vi "BDSCTRL_Main.vi"() -> ()   [LabVIEW 2016]
uses:
  BDSCTRL_Controls/BDSCTRL_Panel_Action_List.ctl
  BDSCTRL_Controls/BDSCTRL_Panel_Poll_Function_List.ctl
  BDSCTRL_Globals/BDSCTRL_Global_Working_Directory.vi
panel:
  in  "error in \n(no error)":errorcluster
  out "Working Directory":path
  in  "stop":bool
  in  "Digital Gain":dbl
  in  "Test Status":string="Awaiting User Selection..."
  in  "Tab Control":T1(tab)
  in  "DMA Settings Cluster":T2
  in  "MB-CFR Settings Cluster":T3
  in  "Set Beam Settings Cluster":T4
  in  "RF Parameters Settings Cluster":T5={"RF Bandwidth \n(MHz)"=0, "Tx RF \nFrequency"=2132.5, "Tx VGA"=[], "Rx VGA"=[]}
  in  "Target Devices":T6={"P1 Cluster"={"P1_D1"=TRUE, "P1_D2"=TRUE, "P1_D3"=TRUE, "P1_D4"=TRUE, "P1_D5"=TRUE, "P1_D6"=TRUE, "P1_D7"=TRUE, "P1_D8"=TRUE, "P1_D9"=TRUE, "P1_D10"=TRUE, "P1_D11"=TRUE, "P1_D12"=TRUE, "P1_D13"=TRUE, "P1_D14"=TRUE, "P1_D15"=TRUE, "P1_D16"=TRUE, "P1_D17"=TRUE, "P1_D18"=TRUE, "P1_D19"=TRUE, "P1_D20"=TRUE, "P1_D21"=TRUE, "P1_D22"=TRUE, "P1_D23"=TRUE, "P1_D24"=TRUE}, "P2 Cluster"={"P2_D1"=TRUE, "P2_D2"=TRUE, "P2_D3"=TRUE, "P2_D4"=TRUE, "P2_D5"=TRUE, "P2_D6"=TRUE, "P2_D7"=TRUE, "P2_D8"=TRUE, "P2_D9"=TRUE, "P2_D10"=TRUE, "P2_D11"=TRUE, "P2_D12"=TRUE, "P2_D13"=TRUE, "P2_D14"=TRUE, "P2_D15"=TRUE, "P2_D16"=TRUE, "P2_D17"=TRUE, "P2_D18"=TRUE, "P2_D19"=TRUE, "P2_D20"=TRUE, "P2_D21"=TRUE, "P2_D22"=TRUE, "P2_D23"=TRUE, "P2_D24"=TRUE}}
  in  "Polling Enable":bool
  in  "Polling Functions":T7
  in  "Read Polling Function":bool
  in  "Query Poll Function":T8
  in  "Exe Panel Action":bool
  in  "Panel Action":T9 items=["Panel Init", "RF Calibration", "Rotate Beam", "Set RF Frequency", "Initial Calibrations", "Channel Enable", "IF Calibration", "Sense Power", "Measure Temperature", "Set RF Power Level", "Run DMA", "Set RF Bandwidth", "Set CFR", "Set Beam"]
  in  "Exe Panel Action Sequence":bool
  in  "Panel Action Sequence":T9[](array[typedef]) items=["Panel Init", "RF Calibration", "Rotate Beam", "Set RF Frequency", "Initial Calibrations", "Channel Enable", "IF Calibration", "Sense Power", "Measure Temperature", "Set RF Power Level", "Run DMA", "Set RF Bandwidth", "Set CFR", "Set Beam"]
  in  "Beam Rotation":string[][](table)=[["1"], ["1"], ["1"], ["1"], ["1"], ["1"], ["2"], ["2"], ["2"], ["2"], ["2"], ["2"]]
  in  "Target String":string="{1:24,1:24,[],[]}"
  in  "Update Targets":bool
  in  "Channels Cluster":T10={"TX1"=TRUE, "TX2"=TRUE, "TX3"=FALSE, "TX4"=FALSE, "TXx3"=TRUE, "TXx4"=TRUE, "RX1"=FALSE, "RX2"=FALSE, "RX3"=FALSE, "RX4"=FALSE, "RXx3"=FALSE, "RXx4"=FALSE, "Tx"=TRUE, "Rx"=FALSE}
  in  "Test List Cluster":T11={"Test List"=[{"Test Process"=enum."Sanity Check", "Update Targets 3"=FALSE, "Enable"=TRUE}, {"Test Process"=enum."Power Accuracy", "Update Targets 3"=FALSE, "Enable"=TRUE}, {"Test Process"=enum."ACLR", "Update Targets 3"=FALSE, "Enable"=TRUE}, {"Test Process"=enum."EVM", "Update Targets 3"=FALSE, "Enable"=TRUE}, {"Test Process"=enum."Rx Sensitivity", "Update Targets 3"=FALSE, "Enable"=TRUE}, {"Test Process"=enum."Scan Beam", "Update Targets 3"=FALSE, "Enable"=TRUE}], "Execute List"=FALSE, "RF Settings List"=[{"RF Bandwidth \n(MHz)"=10, "Tx Frequency \n(MHz)"=2115.0, "TX Attenuation"=[51, 51, 51, 51], "RX Attenuation"=[20, 20, 20, 20], "RF Settings List: Channel Cluster"={"TX1 2"=TRUE, "TX1 3"=TRUE, "TX1 4"=FALSE, "TX1 5"=FALSE, "TX1 6"=TRUE, "TX1 7"=TRUE, "TX1"=FALSE, "TX1 8"=FALSE, "TX1 9"=FALSE, "TX1 10"=FALSE, "TX1 11"=FALSE, "TX1 12"=FALSE, "Tx"=TRUE, "Rx"=FALSE}}, {"RF Bandwidth \n(MHz)"=10, "Tx Frequency \n(MHz)"=2132.5, "TX Attenuation"=[63, 63, 63, 63], "RX Attenuation"=[63, 63, 63, 63], "RF Settings List: Channel Cluster"={"TX1 2"=TRUE, "TX1 3"=TRUE, "TX1 4"=FALSE, "TX1 5"=FALSE, "TX1 6"=TRUE, "TX1 7"=TRUE, "TX1"=FALSE, "TX1 8"=FALSE, "TX1 9"=FALSE, "TX1 10"=FALSE, "TX1 11"=FALSE, "TX1 12"=FALSE, "Tx"=TRUE, "Rx"=FALSE}}]}
  in  "Configure Manual Test":bool
  in  "Test Process":T12(ring)=enum."Scan Beam"
  in  "Execute Test":bool
  in  "Save Settings":bool
  in  "Load Settings":bool
  in  "MXG Test Connection":bool
  in  "EXA Test Connection":bool
  in  "Melvitron Test Connection":bool
  in  "Panel IP Address":string="10.1.11.247"
  in  "EXA IP Address":string="10.1.11.123"
  in  "MXG IP Address":string="10.1.11.122"
  in  "Melvitron IP Address":string="COM12"
  in  "Panel Test Connection":bool
  in  "Test Setup Settings Cluster":T13={"IF Calibration File"=path "IFCalExample.csv", "Beam Lookup Table"=path "BeamLookupTableExample.csv", "Test Environment"=enum."Melvitron", "Panel Mode"=enum."CPRI", "Calibration Mode"=0, "Panel Type"=0, "Band"=0, "Tile"=0, " API Drop"=0} {"API Drop" items=["MAY", "JUNE"]; "Tile" items=["HP-C", "HP-B3"]; "Band" items=["AWS", "PCS-A", "PCS-G"]; "Panel Type" items=["Half", "Full", "Quarter"]; "Calibration Mode" items=["Manual", "SemiAuto", "Auto"]}
  out "SW Version":string
  # "Most useful Panel Status info in common region"
  # "Panel Selections"
  # "Panel Action Settings"
  # "Polling Functions"
  # "Panel Action Execution"
  # "DMA"
  # "MB-CFR"
  # "Set Beam"
  # "RF Parameters"
  # "P2"
  # "P1"
  # "Auto Polling"
  # "Period (s)"
  # "Manual Polling"
  # "Manual Test Process"
  # "Test Connection"
  # "Similar to Panel Status GUI/Window"
  # "Show Results summary from each completed test"
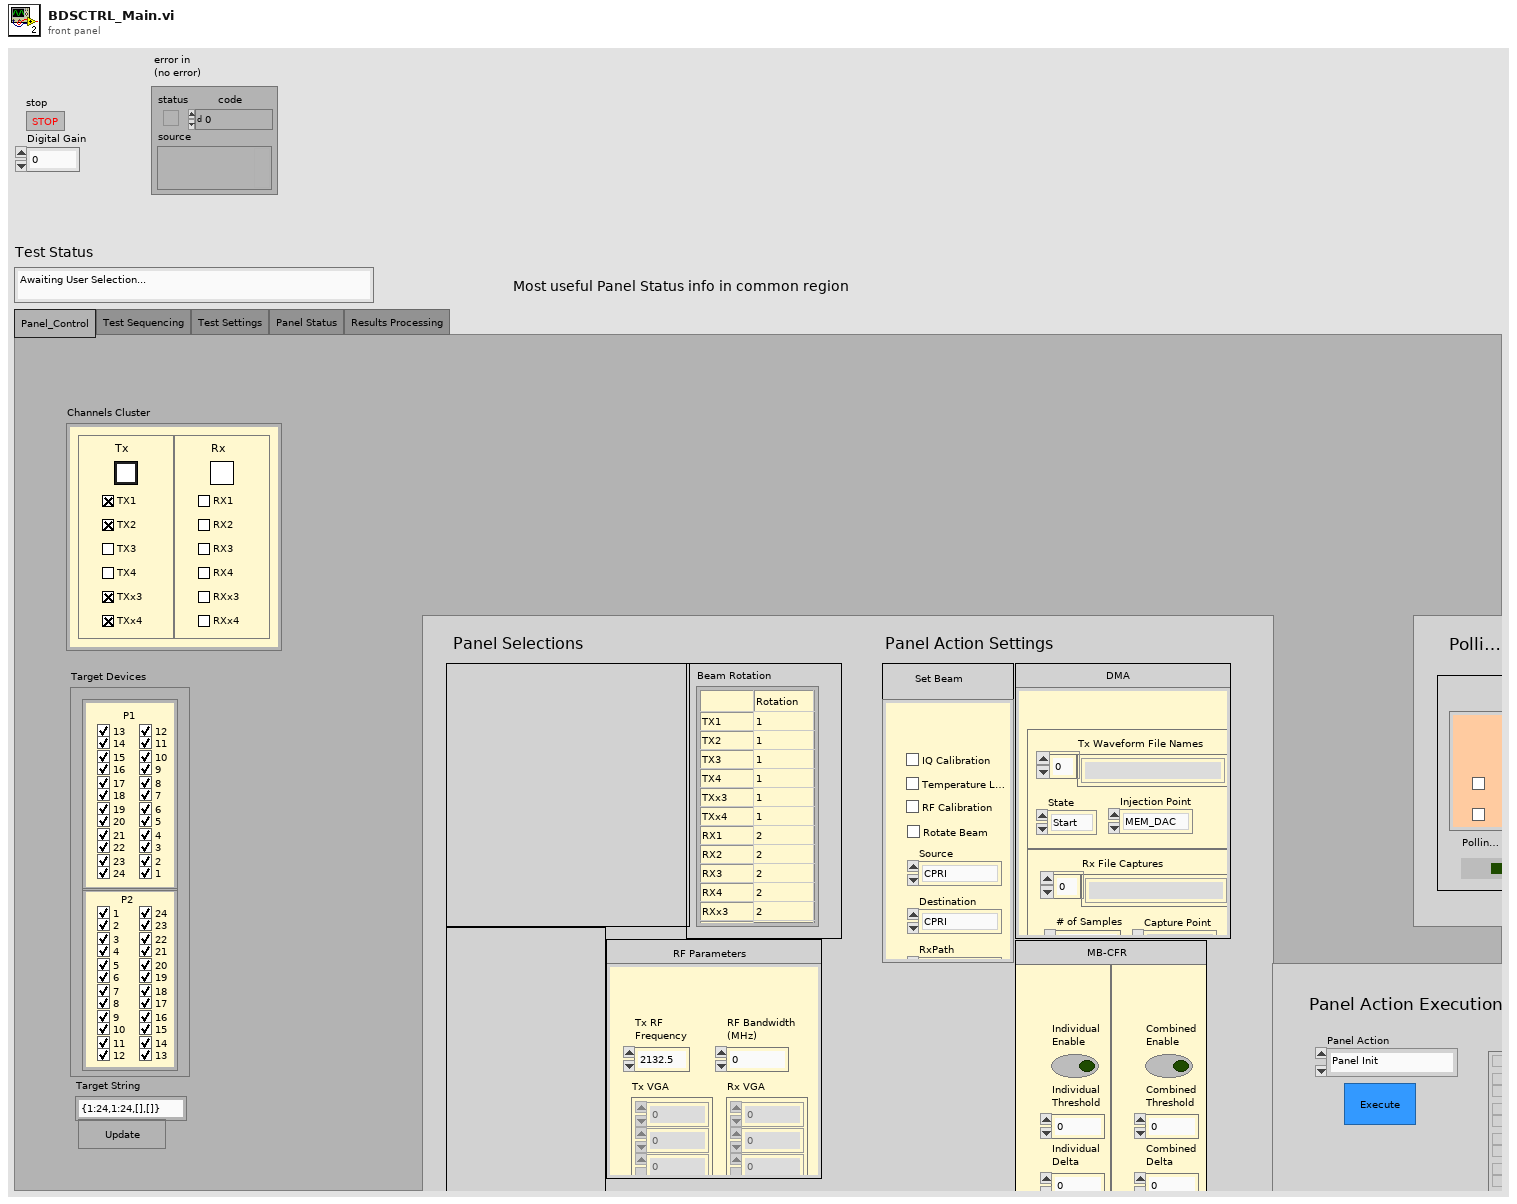
[diagram p1: front panel]
types:
  T1 = enum32{"Panel_Control", "Test Sequencing", "Test Settings", "Panel Status", "Results Processing"}
  T2 = cluster{"Tx Waveform File Names":string[], "State":enum16{"Start", "Stop"}, "Injection Point":enum16{"MEM_DAC", "MEM_DUC"}, "Rx File Captures":string[], "# of Samples":i32, "Capture Point":enum16{"MEM_ADC", "MEM_DDC"}}
  T3 = cluster{"Individual\nEnable":bool, "Individual\nThreshold":dbl, "Individual\nDelta":dbl, "Individual\nWeight":dbl, "Combined\nEnable":bool, "Combined\nThreshold":dbl, "Combined\nDelta":dbl}
  T4 = cluster{"IQ Calibration":bool, "Temperature Loop":bool, "RF Calibration":bool, "Rotate Beam":bool, "Source":enum16{"CPRI", "CAL", "MEM_DAC", "MEM_DUC", "EXT"}, "Destination":enum16{"CPRI", "EXT", "MEM_ADC", "MEM_DDC"}, "RxPath":enum16{"DIRECT", "MIXER"}}
  T5 = cluster{"RF Bandwidth \n(MHz)":i32, "Tx RF \nFrequency":dbl, "Tx VGA":i32[], "Rx VGA":i32[]}
  T6 = cluster{"P1 Cluster":cluster{"P1_D1":bool, "P1_D2":bool, "P1_D3":bool, "P1_D4":bool, "P1_D5":bool, "P1_D6":bool, "P1_D7":bool, "P1_D8":bool, "P1_D9":bool, "P1_D10":bool, "P1_D11":bool, "P1_D12":bool, "P1_D13":bool, "P1_D14":bool, "P1_D15":bool, "P1_D16":bool, "P1_D17":bool, "P1_D18":bool, "P1_D19":bool, "P1_D20":bool, "P1_D21":bool, "P1_D22":bool, "P1_D23":bool, "P1_D24":bool}, "P2 Cluster":cluster{"P2_D1":bool, "P2_D2":bool, "P2_D3":bool, "P2_D4":bool, "P2_D5":bool, "P2_D6":bool, "P2_D7":bool, "P2_D8":bool, "P2_D9":bool, "P2_D10":bool, "P2_D11":bool, "P2_D12":bool, "P2_D13":bool, "P2_D14":bool, "P2_D15":bool, "P2_D16":bool, "P2_D17":bool, "P2_D18":bool, "P2_D19":bool, "P2_D20":bool, "P2_D21":bool, "P2_D22":bool, "P2_D23":bool, "P2_D24":bool}}
  T7 = cluster{"Boolean 6":bool, "Boolean 7":bool, "Boolean 9":bool, dbl, dbl, dbl}
  T8 = typedef "BDSCTRL_Panel_Poll_Function_List.ctl" = enum16{"DFE Info", "DFE Electrical", "DFE Clock", "DFE CPRI", "DFE Temp", "DFE RF Power", "Tile Temperature", "Tile SPI", "Tile Info", "Tile RF Power", "Tile PLL Lock", "Tile PA Linearization", "Tile PA Bias"}
  T9 = typedef "BDSCTRL_Panel_Action_List.ctl" = u16
  T10 = cluster{"TX1":bool, "TX2":bool, "TX3":bool, "TX4":bool, "TXx3":bool, "TXx4":bool, "RX1":bool, "RX2":bool, "RX3":bool, "RX4":bool, "RXx3":bool, "RXx4":bool, "Tx":bool, "Rx":bool}
  T11 = cluster{"Test List":cluster{"Test Process":enum16{"Set Beam", "Scan Beam", "Sanity Check", "Power Accuracy", "ACLR", "EVM", "Rx Sensitivity"}, "Update Targets 3":bool, "Enable":bool}[], "Execute List":bool, "RF Settings List":cluster{"RF Bandwidth \n(MHz)":i32, "Tx Frequency \n(MHz)":dbl, "TX Attenuation":i32[], "RX Attenuation":i32[], "RF Settings List: Channel Cluster":cluster{"TX1 2":bool, "TX1 3":bool, "TX1 4":bool, "TX1 5":bool, "TX1 6":bool, "TX1 7":bool, "TX1":bool, "TX1 8":bool, "TX1 9":bool, "TX1 10":bool, "TX1 11":bool, "TX1 12":bool, "Tx":bool, "Rx":bool}}[]}
  T12 = enum16{"Set Beam", "Scan Beam", "Sanity Check", "Power Accuracy", "ACLR", "EVM", "Rx Sensitivity"}
  T13 = cluster{"IF Calibration File":path, "Beam Lookup Table":path, "Test Environment":enum16{"Melvitron", "Spider", "Marinotron"}, "Panel Mode":enum16{"CPRI", "UpDnCnv"}, "Calibration Mode":u16, "Panel Type":u16, "Band":u16, "Tile":u16, " API Drop":u16}
  T14 = cluster{"Target Devices":cluster{"P1 Cluster":cluster{"P1_D1":bool, "P1_D2":bool, "P1_D3":bool, "P1_D4":bool, "P1_D5":bool, "P1_D6":bool, "P1_D7":bool, "P1_D8":bool, "P1_D9":bool, "P1_D10":bool, "P1_D11":bool, "P1_D12":bool, "P1_D13":bool, "P1_D14":bool, "P1_D15":bool, "P1_D16":bool, "P1_D17":bool, "P1_D18":bool, "P1_D19":bool, "P1_D20":bool, "P1_D21":bool, "P1_D22":bool, "P1_D23":bool, "P1_D24":bool}, "P2 Cluster":cluster{"P2_D1":bool, "P2_D2":bool, "P2_D3":bool, "P2_D4":bool, "P2_D5":bool, "P2_D6":bool, "P2_D7":bool, "P2_D8":bool, "P2_D9":bool, "P2_D10":bool, "P2_D11":bool, "P2_D12":bool, "P2_D13":bool, "P2_D14":bool, "P2_D15":bool, "P2_D16":bool, "P2_D17":bool, "P2_D18":bool, "P2_D19":bool, "P2_D20":bool, "P2_D21":bool, "P2_D22":bool, "P2_D23":bool, "P2_D24":bool}}, "Target String":string}
  T15 = cluster{"Tx RF \nFrequency":dbl, "RF Bandwidth \n(MHz)":i32, "Tx VGA":i32[], "Rx VGA":i32[]}
  T16 = cluster{"Panel IP Address":string, "Melvitron IP Address":string, "EXA IP Address":string, "MXG IP Address":string}
  T17 = cluster{"IF Calibration File":path, "Beam Lookup Table":path, "Test Environment":enum16{"Melvitron", "Spider", "Marinotron"}, "Panel Mode":enum16{"CPRI", "UpDnCnv"}, "Calibration Mode":u16, "Panel Type":u16, "Band":u16, "Tile":u16, "API Drop":u16}
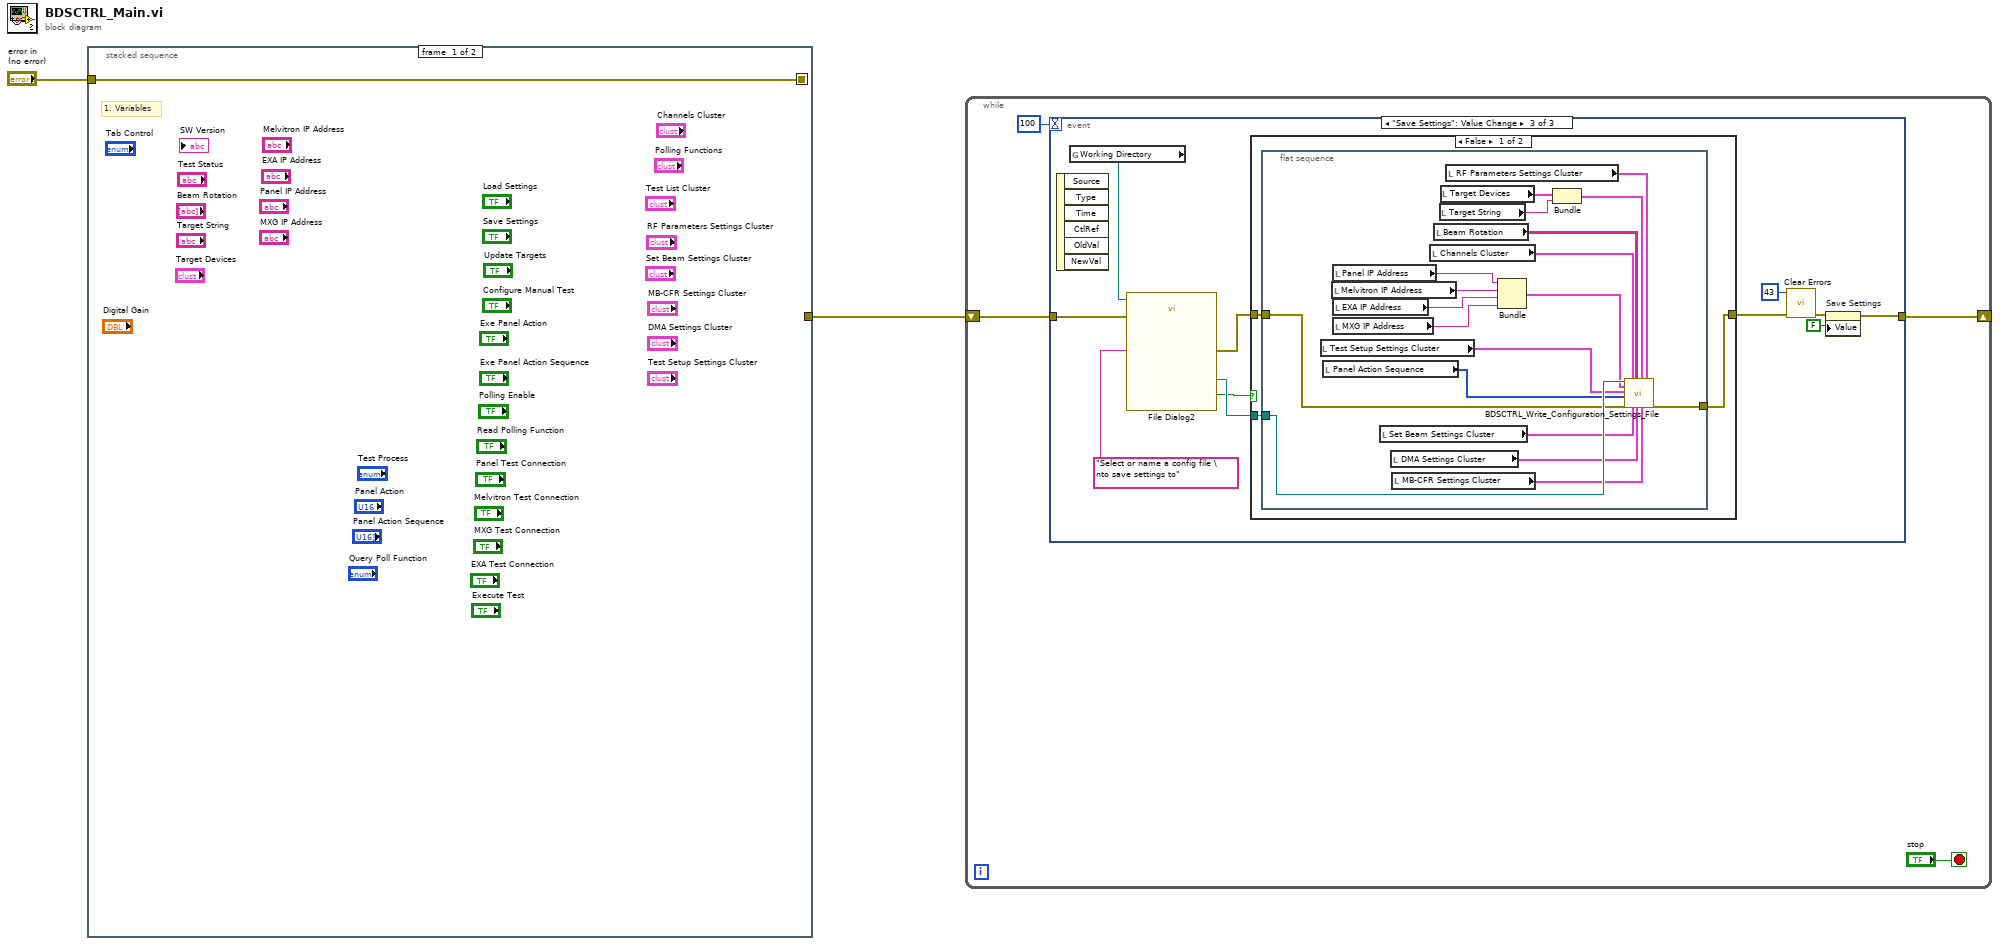
[diagram p0: block diagram]
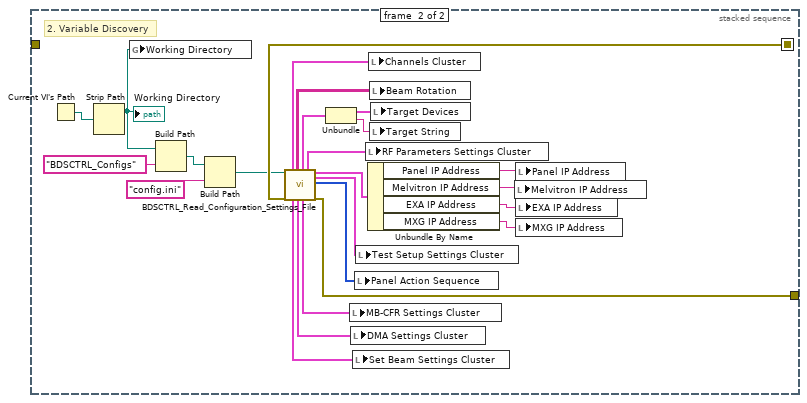
[diagram p2: hidden frame]
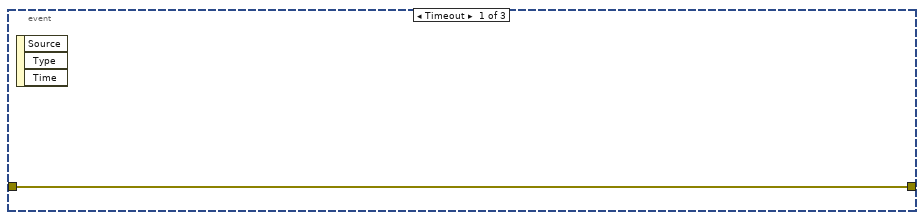
[diagram p3: hidden frame]
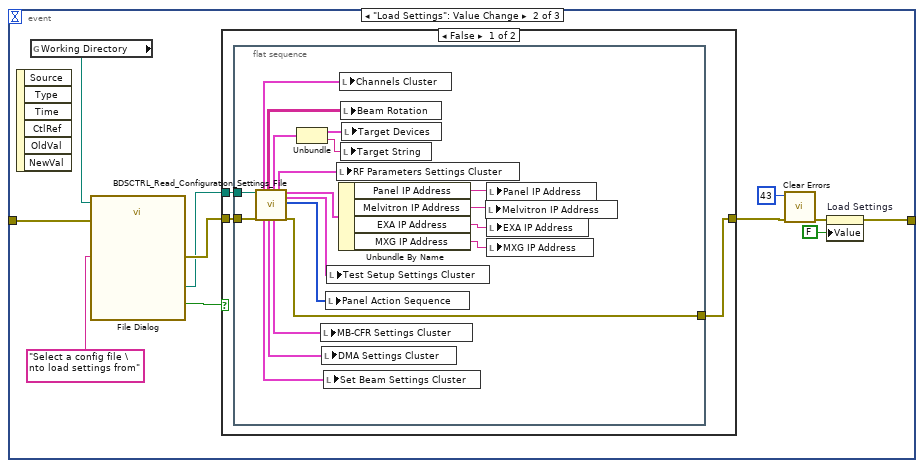
[diagram p4: hidden frame]
diagram:
  n1 = stacked-sequence {
    seq-local: [w3 _] -> [_ w26]
    tunnel: "error in \n(no error)" -> [w3 _]
    tunnel: [_ w6] -> w1
    frame #0 {
      # "1. Variables"
    }
    frame #1 {
      # "2. Variable Discovery"
      n2 = Current VI's Path() -> (path=w27:path)
      n3 = Strip Path(path=w27) -> (stripped path=w25:path)  [unwired: 1 out]
      "Working Directory" <- w25
      n4 = global write "BDSCTRL_Global_Working_Directory.vi" "Working Directory"(w25) -> ()
      n5 = Build Path(base path=w25, name or relative path="BDSCTRL_Configs") -> (appended path=w23:path)
      n6 = Build Path(base path=w23, name or relative path="config.ini") -> (appended path=w21:path)
      n7 = call "BDSCTRL_Read_Configuration_Settings_File.vi"("configuration file path"=w21, "error in \n(no error)"=w26) -> ("Channels Cluster"=w15:T10, "Set Beam Settings Cluster"=w4:T4, "Beam Rotation"=w19:string[][], "DMA Settings Cluster"=w5:T2, "Target Devices Settings Cluster"=w18:T14, "MB-CFR Settings Cluster"=w7:T3, "RF Parameters Settings Cluster"=w20:T15, "BDSCTRL Connection Settings"=w14:T16, "Test Setup Settings"=w9:T17, "Panel Action Sequence"=w8:T9[], "error out"=w6:errorcluster)  [unwired: 7 in]
      n8 = Unbundle(w18) -> ("Target Devices"=w17:T6, "Target String"=w16:string)
      n9 = local write "MB-CFR Settings Cluster"(w7) -> ()
      n10 = local write "DMA Settings Cluster"(w5) -> ()
      n11 = local write "Set Beam Settings Cluster"(w4) -> ()
      n12 = local write "Panel Action Sequence"(w8) -> ()
      n13 = local write "Test Setup Settings Cluster"(w9) -> ()
      n14 = local write "RF Parameters Settings Cluster"(w20) -> ()
      n15 = Unbundle By Name(w14) -> ("Panel IP Address"=w13:string, "Melvitron IP Address"=w12:string, "EXA IP Address"=w11:string, "MXG IP Address"=w10:string)
      n16 = local write "Channels Cluster"(w15) -> ()
      n17 = local write "Beam Rotation"(w19) -> ()
      n18 = local write "Target String"(w16) -> ()
      n19 = local write "Target Devices"(w17) -> ()
      n20 = local write "Melvitron IP Address"(w12) -> ()
      n21 = local write "Panel IP Address"(w13) -> ()
      n22 = local write "EXA IP Address"(w11) -> ()
      n23 = local write "MXG IP Address"(w10) -> ()
    }
  }
  n24 = while {
    shift-right: [w28] -> _
    shift-left: w1 -> [w29]
    stop <- "stop" stop-if-true
    n25 = event shown="[2] \"Save Settings\": Value Change" {
      selector: _ -> [_ _ _]
      dyn-events: _ -> [_ _ _]
      timeout: 100 -> [_ _ _]
      tunnel: w29 -> [w32 w39 w73]
      tunnel: [w32 w38 w71] -> w28
      event Timeout {
        n26 = event-data() -> ()  [unwired: 1 in, 3 out]
      }
      event "Load Settings": Value Change {
        n27 = event-data() -> ()  [unwired: 1 in, 6 out]
        n28 = global read "BDSCTRL_Global_Working_Directory.vi" "Working Directory"() -> (w43:path)
        n29 = call "File Dialog"("start path"=w43, "prompt"="Select a config file \nto load settings from", "error in"=w39) -> ("selected path"=w41:path, "cancelled"=w40:bool, "error out"=w42:errorcluster)  [unwired: 9 in, 1 out]
        n30 = case shown="False" w40 {
          tunnel: w42 -> [w46 w66]
          tunnel: w41 -> [w45 _]
          tunnel: [w44 w66] -> w34
          frame False {
            n31 = flat-sequence {
              tunnel: w46 -> [w49]
              tunnel: w45 -> [w48]
              tunnel: [w47] -> w44
              frame #0 {
                n32 = call "BDSCTRL_Read_Configuration_Settings_File.vi"("configuration file path"=w48, "error in \n(no error)"=w49) -> ("Channels Cluster"=w55:T10, "Set Beam Settings Cluster"=w65:T4, "Beam Rotation"=w51:string[][], "DMA Settings Cluster"=w64:T2, "Target Devices Settings Cluster"=w52:T14, "MB-CFR Settings Cluster"=w63:T3, "RF Parameters Settings Cluster"=w50:T15, "BDSCTRL Connection Settings"=w56:T16, "Test Setup Settings"=w61:T17, "Panel Action Sequence"=w62:T9[], "error out"=w47:errorcluster)  [unwired: 7 in]
                n33 = Unbundle(w52) -> ("Target Devices"=w53:T6, "Target String"=w54:string)
                n34 = local write "MB-CFR Settings Cluster"(w63) -> ()
                n35 = local write "DMA Settings Cluster"(w64) -> ()
                n36 = local write "Set Beam Settings Cluster"(w65) -> ()
                n37 = local write "Panel Action Sequence"(w62) -> ()
                n38 = local write "Test Setup Settings Cluster"(w61) -> ()
                n39 = local write "RF Parameters Settings Cluster"(w50) -> ()
                n40 = Unbundle By Name(w56) -> ("Panel IP Address"=w57:string, "Melvitron IP Address"=w58:string, "EXA IP Address"=w59:string, "MXG IP Address"=w60:string)
                n41 = local write "Channels Cluster"(w55) -> ()
                n42 = local write "Beam Rotation"(w51) -> ()
                n43 = local write "Target String"(w54) -> ()
                n44 = local write "Target Devices"(w53) -> ()
                n45 = local write "Melvitron IP Address"(w58) -> ()
                n46 = local write "Panel IP Address"(w57) -> ()
                n47 = local write "EXA IP Address"(w59) -> ()
                n48 = local write "MXG IP Address"(w60) -> ()
              }
            }
          }
          frame True {
          }
        }
        n49 = call <vilib>:"Clear Errors.vi"("error in (no error)"=w34, "specific error code to clear (0: all)"=43) -> ("error out"=w33:errorcluster)  [unwired: 4 in, 1 out]
        n50 = property on="Load Settings" class="Bool (strict)"(error in=w33, "Value"=FALSE ("Load Settings")) -> (error out=w38:errorcluster)  [unwired: 1 in, 1 out]
      }
      event "Save Settings": Value Change {
        n51 = event-data() -> ()  [unwired: 1 in, 6 out]
        n52 = global read "BDSCTRL_Global_Working_Directory.vi" "Working Directory"() -> (w77:path)
        n53 = call "File Dialog2"("start path"=w77, "prompt"="Select or name a config file \nto save settings to", "error in"=w73) -> ("selected path"=w75:path, "cancelled"=w74:bool, "error out"=w76:errorcluster)  [unwired: 9 in, 1 out]
        n54 = case shown="False" w74 {
          tunnel: w76 -> [w80 w100]
          tunnel: w75 -> [w79 _]
          tunnel: [w78 w100] -> w69
          frame False {
            n55 = flat-sequence {
              tunnel: w80 -> [w81]
              tunnel: w79 -> [w88]
              tunnel: [w99] -> w78
              frame #0 {
                n56 = local read "Test Setup Settings Cluster"() -> (w86:T13)
                n57 = local read "Panel Action Sequence"() -> (w85:T9[])
                n58 = local read "Melvitron IP Address"() -> (w97:string)
                n59 = local read "Panel IP Address"() -> (w98:string)
                n60 = local read "EXA IP Address"() -> (w96:string)
                n61 = local read "MXG IP Address"() -> (w95:string)
                n62 = local read "Set Beam Settings Cluster"() -> (w82:T4)
                n63 = local read "DMA Settings Cluster"() -> (w83:T2)
                n64 = local read "MB-CFR Settings Cluster"() -> (w84:T3)
                n65 = local read "Channels Cluster"() -> (w89:T10)
                n66 = local read "Beam Rotation"() -> (w90:string[][])
                n67 = local read "Target String"() -> (w92:string)
                n68 = local read "Target Devices"() -> (w93:T6)
                n69 = local read "RF Parameters Settings Cluster"() -> (w94:T5)
                n70 = Bundle("Panel IP Address"=w98, "Melvitron IP Address"=w97, "EXA IP Address"=w96, "MXG IP Address"=w95) -> (w87:T16)  [unwired: 1 in]
                n71 = Bundle("Target Devices"=w93, "Target String"=w92) -> (w91:T14)  [unwired: 1 in]
                n72 = call "BDSCTRL_Write_Configuration_Settings_File.vi"("configuration file path"=w88, "BDSCTRL Connection Settings"=w87, "Test Setup Settings"=w86, "Panel Action Sequence"=w85, "error in \n(no error)"=w81, "Channels Cluster"=w89, "Set Beam Settings Cluster"=w82, "Beam Rotation"=w90, "DMA Settings Cluster"=w83, "Target Devices Cluster"=w91, "MB-CFR Settings Cluster"=w84, "RF Parameters Settings Cluster"=w94) -> ("error out"=w99:errorcluster)  [unwired: 7 in]
              }
            }
          }
          frame True {
          }
        }
        n73 = call <vilib>:"Clear Errors.vi"("error in (no error)"=w69, "specific error code to clear (0: all)"=43) -> ("error out"=w68:errorcluster)  [unwired: 4 in, 1 out]
        n74 = property on="Save Settings" class="Bool (strict)"(error in=w68, "Value"=FALSE ("Save Settings")) -> (error out=w71:errorcluster)  [unwired: 1 in, 1 out]
      }
    }
  }
